vi "VocmCF_1212.vi"() -> ()   [LabVIEW 2018]
panel:
  in  "Vocm CF(V) CH1":dbl
  in  "Vocm CF(V) CH0":dbl
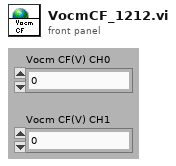
[diagram p1: front panel]
diagram:
